vi "ConfigurationPageConnPane.vi"(9 "Parameter defaults":string, 10 "Parameters":T1, 11 "Stop":T2) -> ()   [LabVIEW 2020, in "ExtensionInterfaces.lvlib" / "IConfigurationPage.lvclass"]
uses:
  IConfigurationPage.lvclass
  Event_StopRef.ctl
  Event_Stop.ctl
  Event_ParametersRef.ctl
  Event_Parameters.ctl
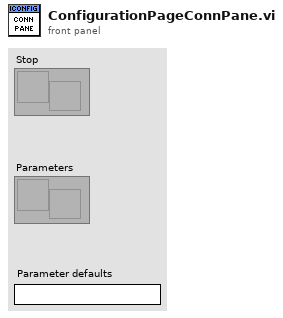
[diagram p1: front panel]
types:
  T1 = typedef "ExtensionInterfaces.lvlib/IConfigurationPage.lvclass/Event_ParametersRef.ctl" = refnum<user-event>
  T2 = typedef "ExtensionInterfaces.lvlib/IConfigurationPage.lvclass/Event_StopRef.ctl" = refnum<user-event>
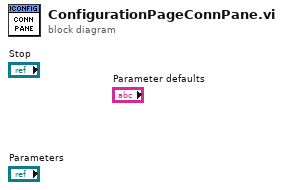
[diagram p0: block diagram]
diagram:
